vi "Set Verbose Linker Errors.vi"(8 "error in (no error)":errorcluster, 10 "Verbose Linker Errors? (true)":bool=TRUE, 11 "DLL in":refnum<class "NI_AB_API_DLL.lvclass">) -> (0 "error out":errorcluster, 3 "DLL out":refnum<class "NI_AB_API_DLL.lvclass">)   [LabVIEW 2020, in "NI_AB_API_DLL.lvclass"]
uses:
  <vilib>/AppBuilder/AB_API/DLL/NI_AB_API_DLL.lvclass
  <vilib>/AppBuilder/AB_API/Application/NI_AB_API_Application.lvclass
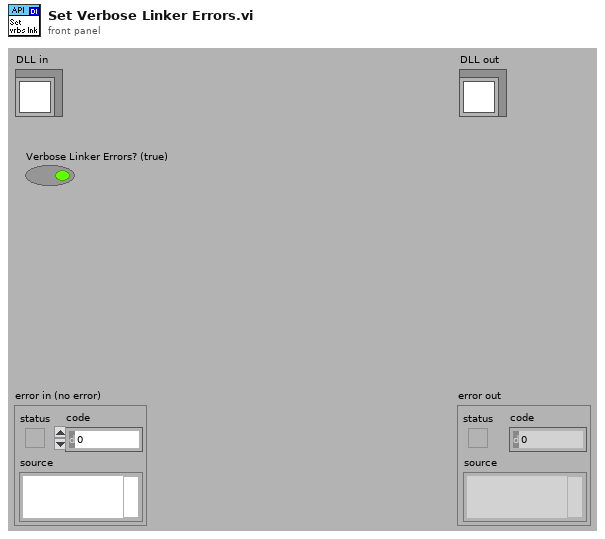
[diagram p1: front panel]
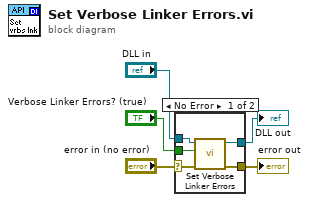
[diagram p0: block diagram]
diagram:
  n1 = case shown="No Error" "error in (no error)" {
    selector: "error in (no error)" -> [w7 w12]
    tunnel: [w8 w12] -> w4
    tunnel: [w9 w11] -> w2
    tunnel: "DLL in" -> [w10 w11]
    tunnel: "Verbose Linker Errors? (true)" -> [w6 _]
    frame No Error {
      n2 = call-parent "Set Verbose Linker Errors.vi"("error in (no error)"=w7, "Verbose Linker Errors? (true)"=w6, "NI_AB_API_Build in"=w10) -> ("error out"=w8:errorcluster, "NI_AB_API_Build out"=w9:refnum<class "NI_AB_API_DLL.lvclass">)  [unwired: 7 in]
    }
    frame Error {
    }
  }
  "error out" <- w4
  "DLL out" <- w2
